vi "Digital Close.vi"(8 "Error In":errorcluster, 10 "Digtal Channel":u8[](array[numeric]), 11 "LINX Resource":T1) -> (0 "Error Out":errorcluster, 3 "LINX Resource":T1)   [LabVIEW 2020, in "LMH-LINX.lvlib"]
doc: "Close the specified digital IO channels."
uses:
  LMH-LINX.lvlib
  Private/Type Defs/LINX Ref.ctl
  Private/Type Defs/Platform.ctl
  Private/Device/Type Defs/LINX Device Config.ctl
  Private/Type Defs/Interface.ctl
  Private/Device/Type Defs/TCP Config.ctl
  Private/Device/Type Defs/Channels.ctl
  Private/Type Defs/Peripheral.ctl
  Private/Type Defs/Error Type.ctl
  Private/myRIO/myRIO.lvlib
  Private/Device/Device.lvlib
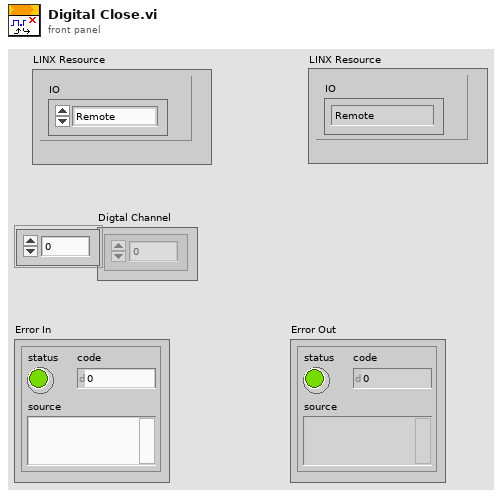
[diagram p1: front panel]
types:
  T1 = typedef "LMH-LINX.lvlib/LINX Ref.ctl" = cluster{"IO":T2, "LINX Device Config":T3}
  T2 = typedef "LMH-LINX.lvlib/Platform.ctl" = enum16{"Remote", "Local"}
  T3 = typedef "Device.lvlib/LINX Device Config.ctl" = cluster{"Interface":T4, "COM Port":refnum<visa-resource-name>, "TCP Configuration":T5, "Device Family":u8, "Device ID":u8, "Device Name":string, "TCP Ref":refnum<k5>, "Channels":T6}
  T4 = typedef "LMH-LINX.lvlib/Interface.ctl" = enum16{"Serial", "TCP"}
  T5 = typedef "Device.lvlib/TCP Config.ctl" = cluster{"IP Address":string, "Port":u16}
  T6 = typedef "LMH-LINX.lvlib/Channels.ctl" = cluster{"DI":u8[], "DO":u8[], "AI":u8[], "AO":u8[], "PWM":u8[], "QE":u8[], "UART":u8[], "I2C 2":u8[], "SPI":u8[], "CAN":u8[], "Servo":u8[], "AI Ref (V)":dbl, "AI Resolution (Bits)":u8, "AO Ref (V)":dbl, "AO Resolution (Bits)":u8}
  T7 = typedef "LMH-LINX.lvlib/Peripheral.ctl" = enum8{"DI", "DO", "AI", "AO", "PWM", "QE", "UART", "I2C", "SPI", "CAN", "Servo"}
  T8 = typedef "LMH-LINX.lvlib/Error Type.ctl" = enum16{"Unknown", "Timeout", "Corrupt Return Packet", "Unable To Connect", "Command Not Supported", "Channel DNE", "Invalid COM Config", "Firmware Version Mismatch", "myRIO Support", "CMD Specific Error", "Local IO Not Supported"}
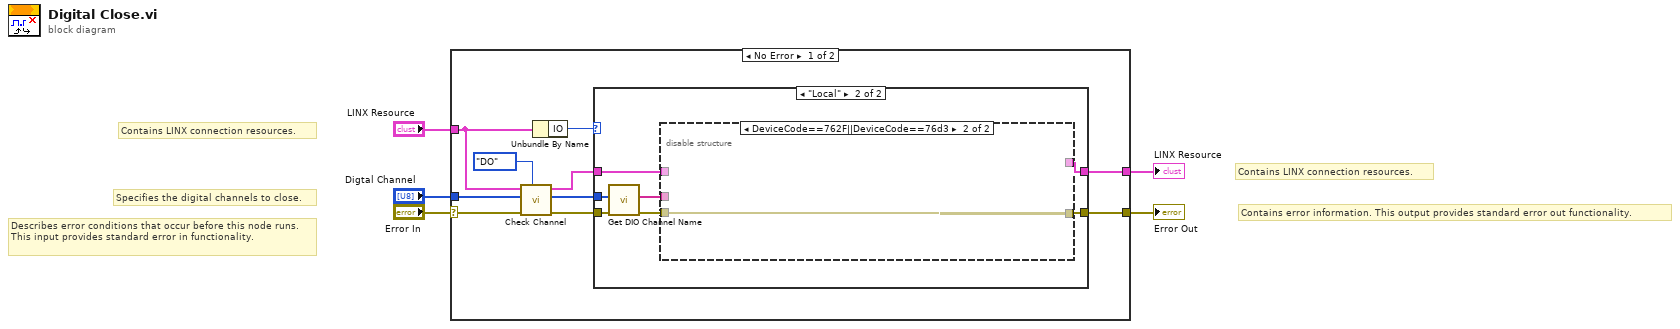
[diagram p0: block diagram]
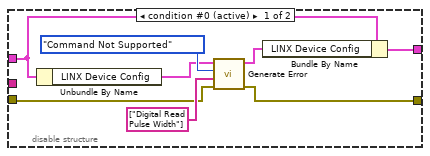
[diagram p3: hidden frame]
diagram:
  # "Specifies the digital channels to close."
  # "Contains LINX connection resources."
  # "Contains error information. This output provides standard error out functionality."
  # "Contains LINX connection resources."
  # "Describes error conditions that occur before this node runs. This input provides standard error in functionality."
  n1 = case shown="No Error" "Error In" {
    selector: "Error In" -> [w6 w35]
    tunnel: [w14 w35] -> w5
    tunnel: [w13 w34] -> w4
    tunnel: "Digtal Channel" -> [w7 _]
    tunnel: "LINX Resource" -> [w8 w34]
    frame No Error {
      n2 = call "Check Channel.vi"("Peripheral"=Peripheral."DO", "Error In"=w6, "Channels"=w7, "LINX Resource"=w8) -> ("Error Out"=w10:errorcluster, "Channels"=w11:u8[], "LINX Resource"=w9:T1)  [unwired: 5 in]
      n3 = Unbundle By Name(w8) -> ("IO"=w15:T2)
      n4 = case shown="\"Local\"" w15 {
        tunnel: w10 -> [w17 w23]
        tunnel: [w17 w20] -> w14
        tunnel: w11 -> [_ w24]
        tunnel: [w16 w19] -> w13
        tunnel: w9 -> [w16 w18]
        frame "Remote", Default {
          # "!!! Send Close Command (Some LINX Devices Might Have A Use For This)"
        }
        frame "Local" {
          n5 = call "Get DIO Channel Name.vi"("Error In"=w23, "DIO Channel Nums"=w24) -> ("Error Out"=w21:errorcluster, "DIO Channels"=w22:string[])  [unwired: 8 in]
          n6 = disable-structure shown="DeviceCode==762F||DeviceCode==76d3" {
            disable-tunnel: w22 -> [_ _]
            disable-tunnel: w21 -> [w27 w33]
            disable-tunnel: [w28 w33] -> w20
            disable-tunnel: [w26 _] -> w19
            disable-tunnel: w18 -> [w25 _]
            frame condition #0 (active) {
              n7 = Unbundle By Name(w25) -> ("LINX Device Config"=w31:T3)
              n8 = call "Generate Error.vi"("Error In"=w27, "Arguments"=string[] ["Digital Read Pulse Width"], "Error Type"=Error_Type."Command Not Supported", "LINX Device Config"=w31) -> ("Error Out"=w28:errorcluster, "Dup LINX Device Config"=w30:T3)  [unwired: 6 in]
              n9 = Bundle By Name(cluster=w25, "LINX Device Config"=w30) -> (w26:T1)
            }
            frame condition #1 {
            }
          }
        }
      }
    }
    frame Error {
    }
  }
  "Error Out" <- w5
  "LINX Resource" <- w4
